vi "XIPIN_IBERT_Virtex5_GTX_(ChipScope_Pro_-_IBERT)_2_01_a.vi"   [LabVIEW 2017]
doc: "The ChipScope(TM) Pro Integrated Bit Error Ratio Tester (IBERT) core for Virtex(R)-5 GTX is a customizable core that can be used to evaluate and monitor the health of Virtex-5 GTX Transceivers.\n------------------------------------\n<b>Need License</b> : No"
uses:
  <vilib>/rvi/XilinxIP/XIPIN_XNode/niFpgaXIPIN.xnode
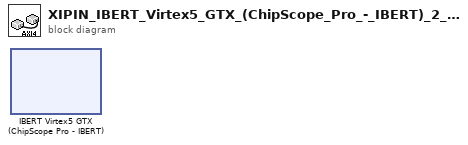
[diagram p0: block diagram]
diagram:
  n1 = xnode ("IBERT Virtex5 GTX (ChipScope Pro - IBERT)")() -> ()
